vi "CSDB_Config.set number values.vi"(2 "Type":string, 3 "Attribute":string, 10 "Values in":string[](array[string]), 12 "InstanceNames":string[](array[string])) -> (16 "Values out":string[](array[string]))   [LabVIEW 2014, in "CSDB_Config.lvlib"]
doc: "sets number values of attribute data"
uses:
  CSDB_Config.lvlib
panel:
  in  "cancel":bool
  in  "apply":bool
  in  "Table":i32[](listbox)
  in  "OK Button":bool
  in  "increment":dbl
  in  "first value":dbl
  # "u - unsigned\ni   - integer\nd - double\n(All values are written\nwith double precision)"
  # "Set Values"
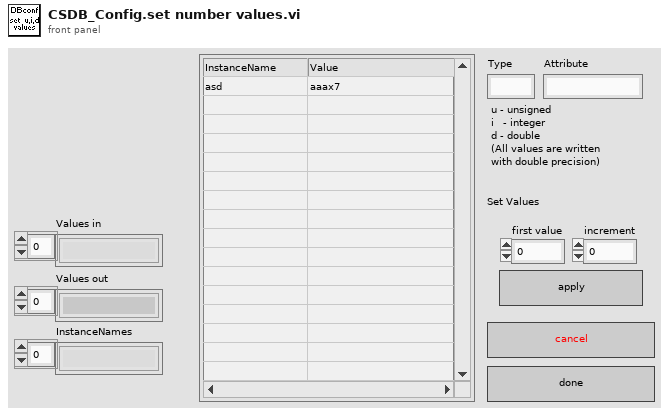
[diagram p1: front panel]
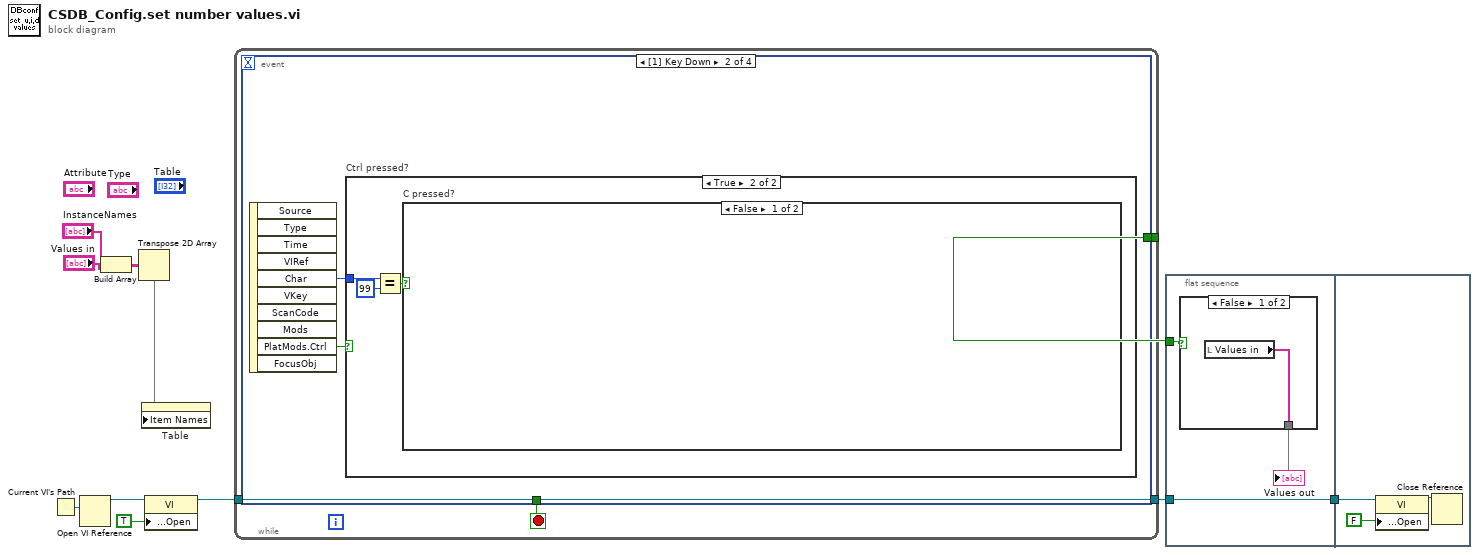
[diagram p0: block diagram]
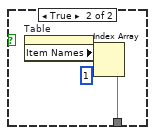
[diagram p2: hidden frame]
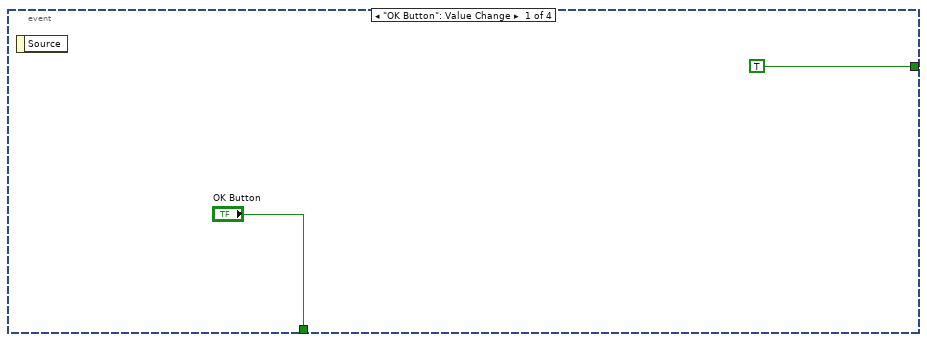
[diagram p3: hidden frame]
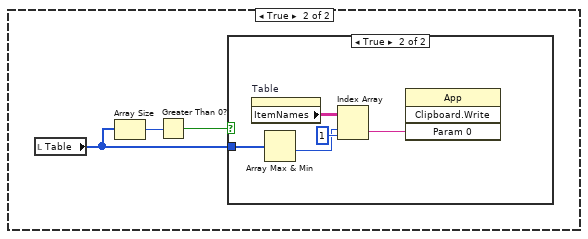
[diagram p5: hidden frame]
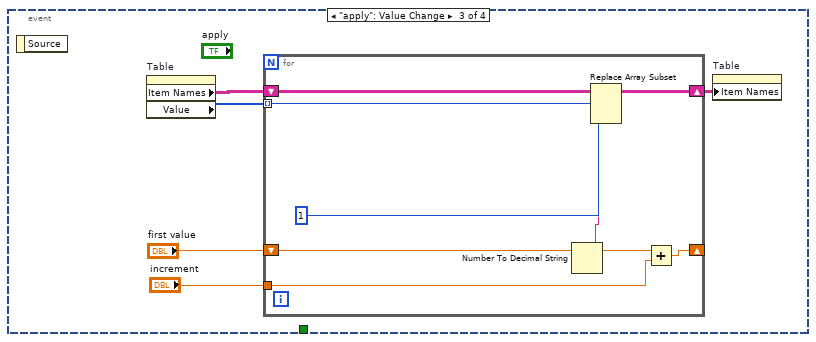
[diagram p7: hidden frame]
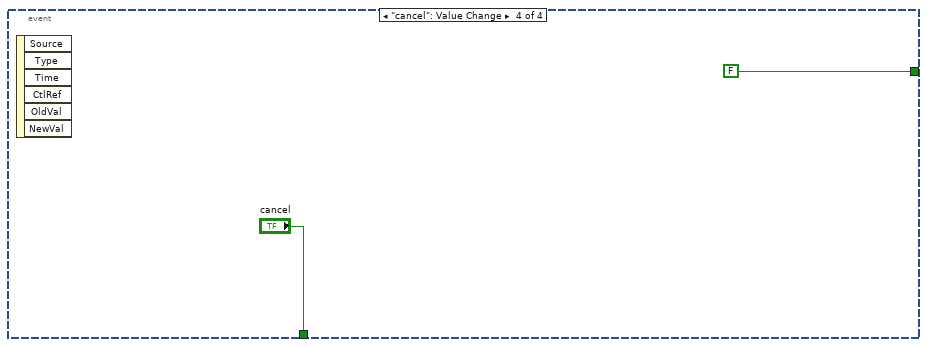
[diagram p8: hidden frame]
diagram:
  n1 = Current VI's Path() -> (path=w11:path)
  n2 = Open VI Reference(vi path=w11) -> (vi reference=w10:refnum<vi>)  [unwired: 5 in, 1 out]
  n3 = Build Array("InstanceNames", "Values in") -> (w4:string[][])
  n4 = Transpose 2D Array(2D array=w4) -> (transposed array=w3:string[][])
  n5 = property on="Table" class="MCListbox (strict)"("Item Names"=w3) -> ()  [unwired: 2 in, 2 out]
  n6 = property class="VI"(reference=w10, "Front Panel Window:Open"=TRUE) -> (reference out=w8:refnum<vi>)  [unwired: 1 in, 1 out]
  n7 = while {
    tunnel: [w14] -> w7
    tunnel: w8 -> [w14]
    tunnel: [w12] -> w1
    stop <- w13 stop-if-true
    n8 = event shown="[1] Key Down" {
      selector: _ -> [_ _ _ _]
      dyn-events: _ -> [_ _ _ _]
      timeout: _ -> [_ _ _ _]
      tunnel: ["OK Button" _ _ "cancel"] -> w13
      tunnel: [TRUE _ _ FALSE] -> w12
      event "OK Button": Value Change {
        n9 = event-data() -> ()  [unwired: 1 in, 1 out]
      }
      event Key Down {
        n10 = event-data() -> ("Char"=w18:i16, "PlatMods.Ctrl"=w17:bool)  [unwired: 1 in, 8 out]
        n11 = case "Ctrl pressed?" shown="True" w17 {
          tunnel: w18 -> [_ w19]
          frame False {
          }
          frame True {
            n12 = Equal?(x=w19, y=i16 99) -> (x = y?=w20:bool)
            n13 = case "C pressed?" shown="False" w20 {
              frame False {
              }
              frame True {
                n14 = local read "Table"() -> (w22:i32[])
                n15 = Array Size(array=w22) -> (size(s)=w24:i32)
                n16 = Greater Than 0?(x=w24) -> (x > 0?=w23:bool)
                n17 = case shown="True" w23 {
                  tunnel: w22 -> [_ w27]
                  frame False {
                  }
                  frame True {
                    n18 = property on="Table" class="MCListbox (strict)"() -> ("ItemNames"=w25:string[][])  [unwired: 2 in, 2 out]
                    n19 = Array Max & Min(array=w27) -> (min value=w26:i32)  [unwired: 3 out]
                    n20 = Index Array(array=w25, index (row)=w26, index (col)=1 ("disabled index (col)")) -> (element=w29:string)
                    n21 = invoke class="App" method="Clipboard.Write"("Param 0"=w29) -> ()  [unwired: 3 in, 4 out]
                  }
                }
              }
            }
          }
        }
      }
      event "apply": Value Change {
        n22 = event-data() -> ()  [unwired: 1 in, 1 out]
        n23 = property on="Table" class="MCListbox (strict)"() -> ("Item Names"=w34:string[][], "Value"=w33:i32[])  [unwired: 2 in, 2 out]
        n24 = for {
          tunnel: w33 -> [w41] mode=indexing
          shift-right: [w38] -> _
          shift-left: "first value" -> [w39]
          tunnel: "increment" -> [w37]
          shift-right: [w36] -> w30
          shift-left: w34 -> [w42]
          n25 = Number To Decimal String(number=w39) -> (decimal integer string=w35:string)  [unwired: 1 in]
          n26 = Replace Array Subset(array=w42, new element=w35, index (row)=w41, index (col)=1 ("disabled index (col)")) -> (w36:string[][])
          n27 = Add(x=w39, y=w37) -> (x+y=w38:dbl)
        }
        n28 = property on="Table" class="MCListbox (strict)"("Item Names"=w30) -> ()  [unwired: 2 in, 2 out]
      }
      event "cancel": Value Change {
        n29 = event-data() -> ()  [unwired: 1 in, 6 out]
      }
    }
  }
  n30 = flat-sequence {
    tunnel: w7 -> [w46]
    tunnel: [w46] -> w2
    tunnel: w1 -> [w45]
    tunnel: w2 -> [w52]
    frame #0 {
      n31 = case shown="False" w45 {
        tunnel: [w48 w49] -> w47
        frame False {
          n32 = local read "Values in"() -> (w48:string[])
        }
        frame True {
          n33 = property on="Table" class="MCListbox (strict)"() -> ("Item Names"=w51:string[][])  [unwired: 2 in, 2 out]
          n34 = Index Array(array=w51, index (col)=1 ("disabled index (col)")) -> (element=w49:string[])  [unwired: 1 in]
        }
      }
      "Values out" <- w47
    }
    frame #1 {
      n35 = property class="VI"(reference=w52, "Front Panel Window:Open"=FALSE) -> (reference out=w54:refnum<vi>)  [unwired: 1 in, 1 out]
      n36 = Close Reference(reference=w54) -> ()  [unwired: 1 in, 1 out]
    }
  }
